vi "AxisAngle to Rotation.vi"(1 "vector":dbl[](array[numeric]), 2 "angle (rad)":dbl, 3 "quaternion":dbl[](array[numeric])) -> (0 "rotation matrix":T1)   [LabVIEW 2024]
uses:
  <vilib>/Analysis/Matrix/Datatypes/RealMatrix.ctl
  <vilib>/Analysis/_algsub.llb/Real Vector Norm.vi
  <vilib>/Analysis/NI_AALPro.lvlib
  <vilib>/Analysis/Matrix/NI_Matrix.lvlib
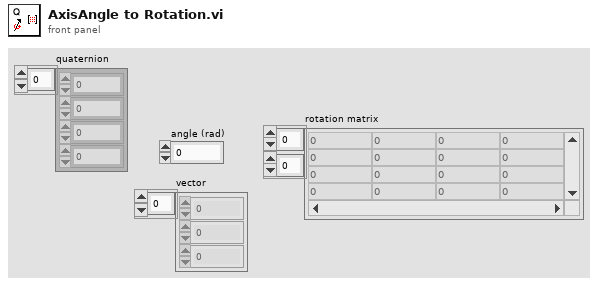
[diagram p1: front panel]
types:
  T1 = typedef "NI_Matrix.lvlib/RealMatrix.ctl" = dbl[][]
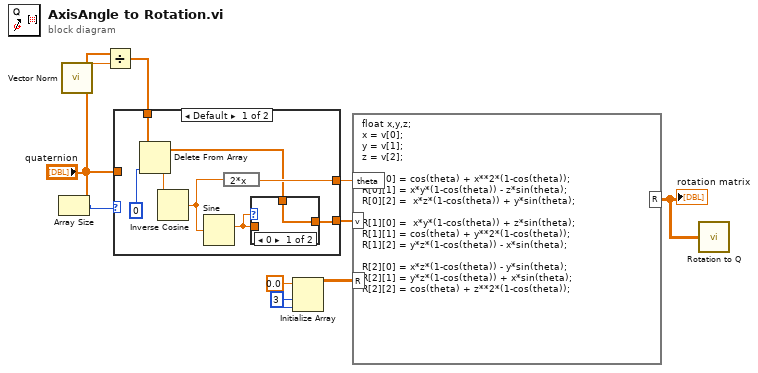
[diagram p0: block diagram]
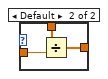
[diagram p2: hidden frame]
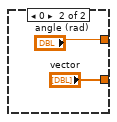
[diagram p3: hidden frame]
diagram:
  w9 = 3 ("dimension size")
  n1 = Array Size(array="quaternion") -> (size(s)=w5:i32)
  n2 = call-poly <vilib>:"Vector Norm.vi"("Input Vector"="quaternion") -> ("norm"=w3:dbl)  [unwired: 9 in, 1 out]
  n3 = Divide(x="quaternion", y=w3) -> (x/y=w2:dbl[])
  n4 = case shown="Default" w5 {
    tunnel: [w13 "vector"] -> w10
    tunnel: [w16 "angle (rad)"] -> w6
    tunnel: "quaternion" -> [_ _]
    tunnel: w2 -> [w12 _]
    frame Default {
      n5 = Delete From Array(array=w12, index=0) -> (deleted portion=w17:dbl, array with subset deleted=w14:dbl[])  [unwired: 1 in]
      n6 = Inverse Cosine(1:w17) -> (0:w15:dbl)
      n7 = Sine(x=w15) -> (sin(x)=w11:dbl)
      n8 = expression code="2*x"(w15) -> (w16:dbl)
      n9 = case shown="0" w11 {
        tunnel: w14 -> [w19 w22]
        tunnel: w11 -> [_ w21]
        tunnel: [w19 w20] -> w13
        frame 0 {
        }
        frame Default {
          n10 = Divide(x=w22, y=w21) -> (x/y=w20:dbl[])
        }
      }
    }
    frame 0 {
    }
  }
  n11 = Initialize Array(0.0 ("element"), w9, w9) -> (w8:dbl[][])
  n12 = formula code="float x,y,z;\nx = v[0];\ny = v[1];\nz = v[2];\n\nR[0][0] = cos(theta) + x**2*(1-cos(theta));\nR[0][1] = x*y*(1-cos(theta)) - z*sin(theta);\nR[0][2] =  x*z*(1-cos(theta)) + y*sin(theta);\n\nR[1][0] =  x*y*(1-cos(theta)) + z*sin(theta);\nR[1][1] = cos(theta) + y**2*(1-cos(theta));\nR[1][2] = y*z*(1-cos(theta)) - x*sin(theta);\n\nR[2][0] = x*z*(1-cos(theta)) - y*sin(theta);\nR[2][1] = y*z*(1-cos(theta)) + x*sin(theta);\nR[2][2] = cos(theta) + z**2*(1-cos(theta));"("v"=w10, "R"=w8, "theta"=w6) -> ("R"=w1:dbl[][])
  "rotation matrix" <- w1
  n13 = call <userlib>:"Rotation to Q.vi"("Rotation matrix"=w1) -> ()  [unwired: 3 out]
